vi "sinlge_motor.vi"() -> ()   [LabVIEW 2023]
uses:
  <vilib>/Python/Open Venv Python Session.vi
  <instrlib>/Phidgets/Phidget Voltage Ratio Input/Public/VoltageRatioInputStart.vi
  <instrlib>/Phidgets/Phidget Voltage Ratio Input/Public/VoltageRatioInputClose.vi
  <instrlib>/Phidgets/Phidget Common/Phidget Common.lvlib
  <instrlib>/Phidgets/Phidget Voltage Ratio Input/Phidget Voltage Ratio Input.lvlib
panel:
  in  "Max Torque":dbl
  in  "Velocity":dbl
  in  "IsHubPort":bool
  out "Serial Number Return":i32
  in  "Device Info":T1={"Serial Number"=-1, "Channel"=0, "Port"=0}
  out "error out":errorcluster
  out "Voltage Ratio":dbl format="%_4g"
  out "Torque":dbl
  in  "Torque":dbl
  in  "Position":dbl
  out "main error":errorcluster
  out "Position":dbl
  in  "Control Selection":T2(ring)
  out "Close session error":errorcluster
  out "start error":errorcluster
  out "iter":dbl
  in  "?":bool
  # "Motor Telemetry"
  # "Motor Controls"
  # "Move Controls"
  # "Load Cell Output"
  # "Velocity Torque Max Controls"
  # "Torque Control"
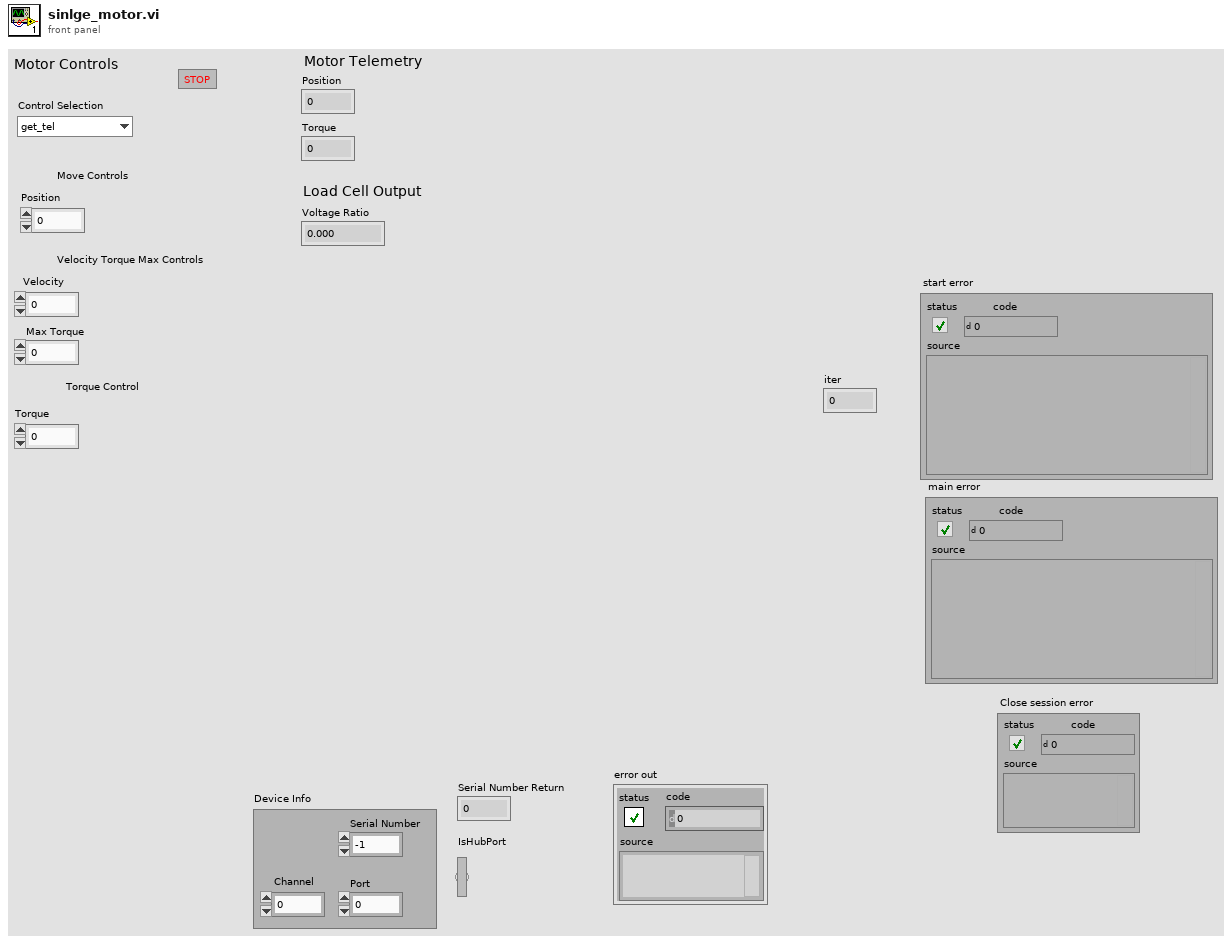
[diagram p1: front panel]
types:
  T1 = cluster{"Serial Number":i32, "Channel":i32, "Port":i32}
  T2 = enum16{"get_tel", "hold", "move", "vel_trq", "torque"}
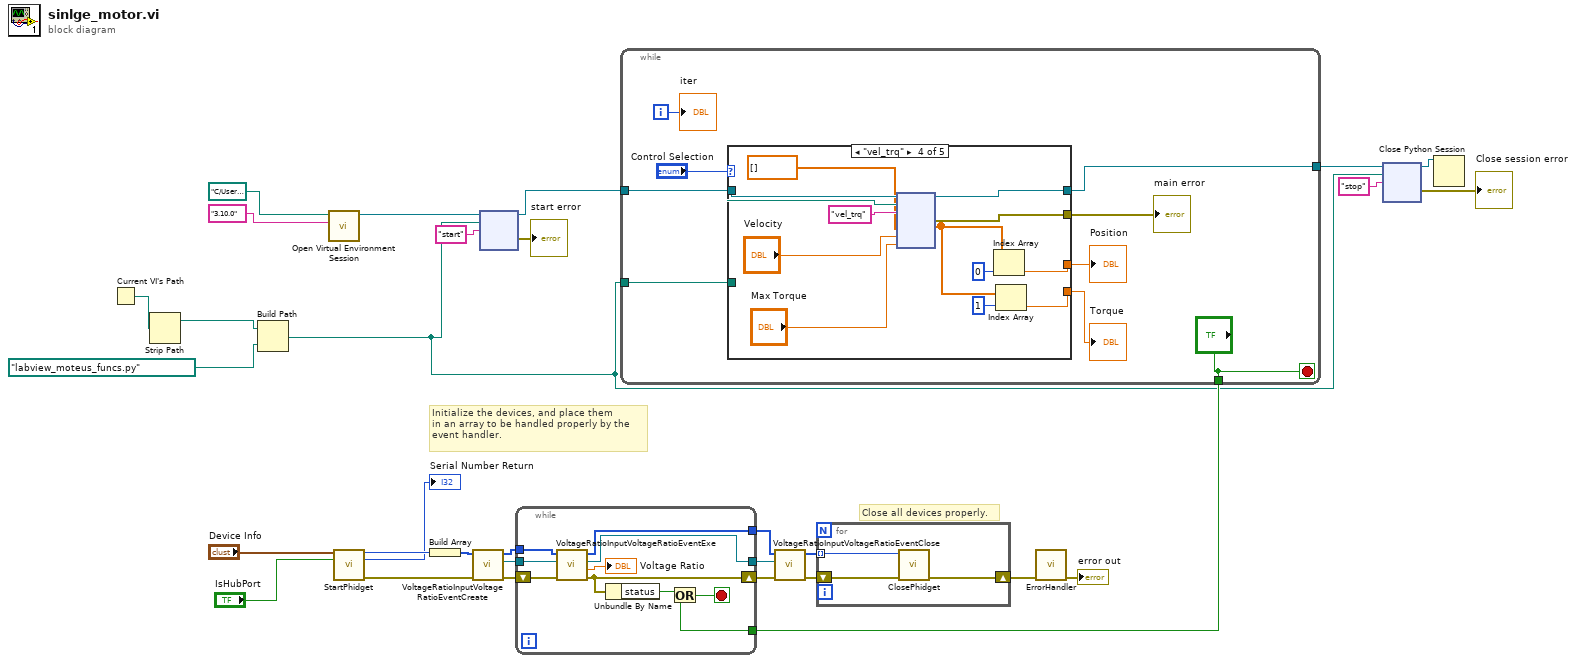
[diagram p0: block diagram]
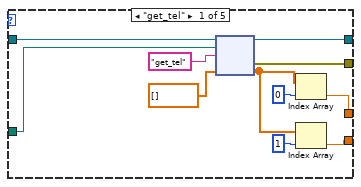
[diagram p2: hidden frame]
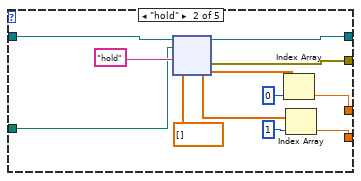
[diagram p3: hidden frame]
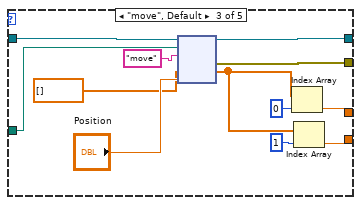
[diagram p4: hidden frame]
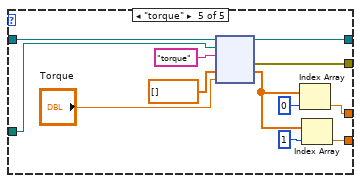
[diagram p5: hidden frame]
diagram:
  # "Close all devices properly."
  # "Initialize the devices, and place them\nin an array to be handled properly by the\nevent handler."
  n1 = Current VI's Path() -> (path=w4:path)
  n2 = Strip Path(path=w4) -> (stripped path=w3:path)  [unwired: 1 out]
  n3 = Build Path(base path=w3, name or relative path=path "labview_moteus_funcs.py") -> (appended path=w1:path)
  n4 = call-poly <vilib>:"Open Virtual Environment Session.vi"("Python version"="3.10.0", "Env path"=path "C:/Users/bjohnst1/Documents/biomech_res/res_env2") -> ("session out"=w27:refnum<k35>)  [unwired: 8 in, 1 out]
  n5 = call-poly <instrlib>:"StartPhidget.vi"("Device Info"="Device Info", "IsHubPort"="IsHubPort") -> ("Phidget ID"=w11:u64, "Serial Number Return"=→"Serial Number Return":i32, "error out"=w7:errorcluster)  [unwired: 10 in, 1 out]
  n6 = Build Array(w11) -> (w21:u64[])
  n7 = call <instrlib>:"VoltageRatioInputVoltageRatioEventCreate.vi"("error in (no error)"=w7, "Devices In"=w21) -> ("error out"=w14:errorcluster, "Event Registration Refnum"=w19:refnum<event-registration>, "Devices Out"=w20:u64[])  [unwired: 7 in]
  n8 = node(w27, w1, "start") -> (w26:refnum<k35>, →"start error":errorcluster)  [unwired: 3 in, 2 out]
  n9 = while {
    tunnel: [w39] -> w25
    tunnel: w26 -> [w38]
    tunnel: w1 -> [w37]
    tunnel: ["?"] -> w5
    i -> [w40]
    stop <- "?" stop-if-true
    n10 = case shown="\"vel_trq\"" "Control Selection" {
      tunnel: [w51 w62 w74 w87 w99] -> w39
      tunnel: w38 -> [w49 w60 w72 w85 w97]
      tunnel: [w48 w59 w70 w83 w96] -> w35
      tunnel: w37 -> [w47 w58 w69 w82 w95]
      tunnel: [w42 w52 w63 w76 w90] -> w34
      tunnel: [w41 w53 w64 w75 w89] -> w33
      frame "get_tel" {
        n11 = node(w49, w47, "get_tel", dbl[] []) -> (w51:refnum<k35>, w48:errorcluster, w43:dbl[])  [unwired: 1 in, 2 out]
        n12 = Index Array(array=w43, index=0) -> (element=w41:dbl)
        n13 = Index Array(array=w43, index=1) -> (element=w42:dbl)
      }
      frame "hold" {
        n14 = node(w60, w58, "hold", dbl[] []) -> (w62:refnum<k35>, w59:errorcluster, w54:dbl[])  [unwired: 1 in, 2 out]
        n15 = Index Array(array=w54, index=0) -> (element=w53:dbl)
        n16 = Index Array(array=w54, index=1) -> (element=w52:dbl)
      }
      frame "move", Default {
        n17 = node(w72, w69, "move", dbl[] [], "Position") -> (w74:refnum<k35>, w70:errorcluster, w65:dbl[])  [unwired: 2 in, 2 out]
        n18 = Index Array(array=w65, index=0) -> (element=w64:dbl)
        n19 = Index Array(array=w65, index=1) -> (element=w63:dbl)
      }
      frame "vel_trq" {
        n20 = node(w85, w82, "vel_trq", dbl[] [], "Velocity", "Max Torque") -> (w87:refnum<k35>, w83:errorcluster, w77:dbl[])  [unwired: 3 in, 2 out]
        n21 = Index Array(array=w77, index=0) -> (element=w75:dbl)
        n22 = Index Array(array=w77, index=1) -> (element=w76:dbl)
      }
      frame "torque" {
        n23 = node(w97, w95, "torque", dbl[] [], "Torque") -> (w99:refnum<k35>, w96:errorcluster, w91:dbl[])  [unwired: 2 in, 2 out]
        n24 = Index Array(array=w91, index=0) -> (element=w89:dbl)
        n25 = Index Array(array=w91, index=1) -> (element=w90:dbl)
      }
    }
    "main error" <- w35
    "Torque" <- w34
    "Position" <- w33
    "iter" <- w40
  }
  n26 = while {
    tunnel: w20 -> [w109]
    tunnel: w19 -> [w105]
    tunnel: [w108] -> w16
    shift-right: [w104] -> w15
    shift-left: w14 -> [w107]
    tunnel: [w106] -> w9
    tunnel: w5 -> [w100]
    stop <- w103 stop-if-true
    n27 = call <instrlib>:"VoltageRatioInputVoltageRatioEventExe.vi"("error in (no error)"=w107, "Event Registration Refnum In"=w105, "Devices In"=w109) -> ("error out"=w104:errorcluster, "VoltageRatio"=→"Voltage Ratio":dbl, "Event Registration Refnum Out"=w108:refnum<event-registration>, "Devices Out"=w106:u64[])  [unwired: 2 in, 3 out]
    n28 = Unbundle By Name(w104) -> ("status"=w102:bool)
    n29 = Or(x=w102, y=w100) -> (x .or. y?=w103:bool)
  }
  n30 = call <instrlib>:"VoltageRatioInputVoltageRatioEventClose.vi"("error in (no error)"=w15, "Event Registration Refnum In"=w16, "Devices In"=w9) -> ("error out"=w12:errorcluster, "Devices Out"=w10:u64[])  [unwired: 7 in]
  n31 = for {
    tunnel: w10 -> [w110] mode=indexing
    shift-right: [w112] -> w18
    shift-left: w12 -> [w111]
    n32 = call-poly <instrlib>:"ClosePhidget.vi"("error in"=w111, "Device In"=w110) -> ("error out"=w112:errorcluster)  [unwired: 9 in]
  }
  n33 = call <instrlib>:"ErrorHandler.vi"("error in"=w18) -> ("error out"=→"error out":errorcluster)  [unwired: 9 in, 1 out]
  n34 = node(w25, w1, "stop") -> (w24:refnum<k35>, →"Close session error":errorcluster)  [unwired: 3 in, 2 out]
  n35 = Close Python Session(session in=w24) -> ()  [unwired: 1 in, 1 out]
